vi "GetKnobType.vi"(8 "error in (no error)":errorcluster, 11 "reference in":refnum<vi>) -> (0 "error out":errorcluster, 2 "Knob Type":string, 3 "reference out":refnum<vi>)   [LabVIEW 2019]
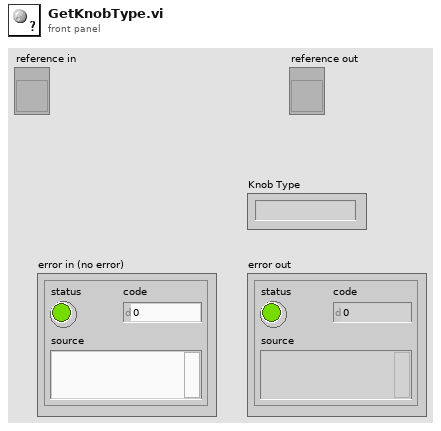
[diagram p1: front panel]
types:
  T1 = typedef "LVNumericRepresentation.ctl" = enum32{"Extended Precision", "Double Precision", "Single Precision", "Long", "Word", "Byte", "Unsigned Long", "Unsigned Word", "Unsigned Byte", "Complex Extended", "Complex Double", "Complex Single", "Quad", "Unsigned Quad", "Fixed-Point"}
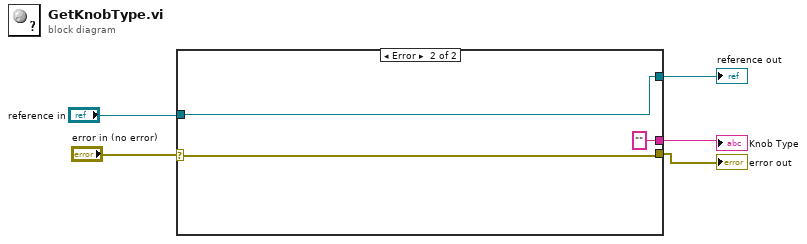
[diagram p0: block diagram]
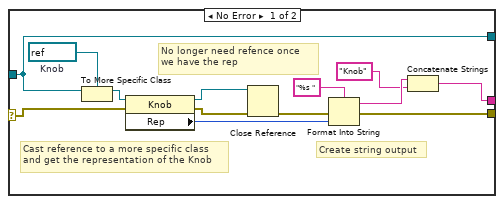
[diagram p2: hidden frame]
diagram:
  n1 = case shown="Error" "error in (no error)" {
    selector: "error in (no error)" -> [w11 w21]
    tunnel: "reference in" -> [w6 w19]
    tunnel: [w8 ""] -> w4
    tunnel: [w9 w21] -> w5
    tunnel: [w6 w19] -> w1
    frame No Error {
      w16 = refnum<vi> refnum  # Knob
      # "Create string output"
      # "No longer need refence once \nwe have the rep"
      # "Cast reference to a more specific class\nand get the representation of the Knob"
      n2 = To More Specific Class(target class=w16, reference=w6) -> (specific class reference=w15:refnum<vi>)  [unwired: 1 in, 1 out]
      n3 = property class="Knob"(reference=w15, error in=w11) -> (reference out=w14:refnum<vi>, error out=w13:errorcluster, "Rep"=w12:T1)
      n4 = Close Reference(reference=w14, error in (no error)=w13) -> (error out=w18:errorcluster)
      n5 = Format Into String(format string="%s ", error in=w18, w12) -> (resulting string=w10:string, error out=w9:errorcluster)  [unwired: 1 in]
      n6 = Concatenate Strings(w10, "Knob" ("string")) -> (w8:string)
    }
    frame Error {
    }
  }
  "error out" <- w5
  "Knob Type" <- w4
  "reference out" <- w1
